vi "LVtoJSON-DBUpdateAll.vi"(0 "Table":string="Inventory", 1 "Update All":bool, 2 "SQL Query Statement":string, 3 "Column Number":i32, 5 "SQL Statement":string, 9 "Reply Command":string="Inventory", 11 "error in":errorcluster, 12 "Payload":string="Inventory", 14 "Datatype":i32) -> (4 "Output JSON Object":string, 15 "error out":errorcluster)   [LabVIEW 2014]
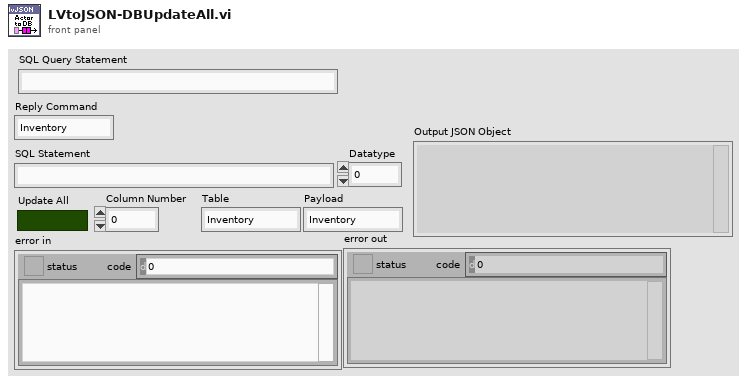
[diagram p1: front panel]
types:
  T1 = cluster{"Table":string, "SQL Statement":string, "Update All":bool, "Payload":string, "Column Number":i32, "Datatype":i32, "Reply Command":string, "SQL Query Statement":string}
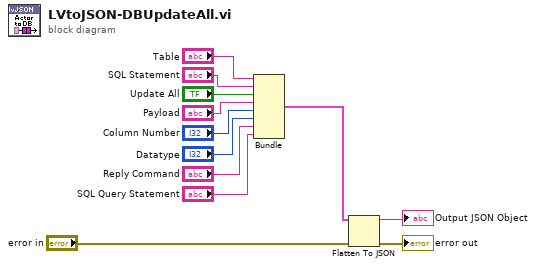
[diagram p0: block diagram]
diagram:
  n1 = Bundle("Table"="Table", "SQL Statement"="SQL Statement", "Update All"="Update All", "Payload"="Payload", "Column Number"="Column Number", "Datatype"="Datatype", "Reply Command"="Reply Command", "SQL Query Statement"="SQL Query Statement") -> (w6:T1)  [unwired: 1 in]
  n2 = Flatten To JSON(anything=w6, error in (no error)="error in") -> (JSON string=→"Output JSON Object":string, 11:→"error out":errorcluster)  [unwired: 1 in]
